vi "daqmx_task output_test.vi"() -> ()   [LabVIEW 2013]
uses:
  <vilib>/DAQmx/read.llb/DAQmx Read (Analog 1D Wfm NChan NSamp).vi
panel:
  out "time string 3":string
  out "time string 2":string
  out "time string":string
  out "error out 2":errorcluster
  out "error out":errorcluster
  out "data 3":waveform(dbl)[](graph) caption="data"
  out "data 2":waveform(dbl)[](graph) caption="data"
  out "data":waveform(dbl)[](graph)
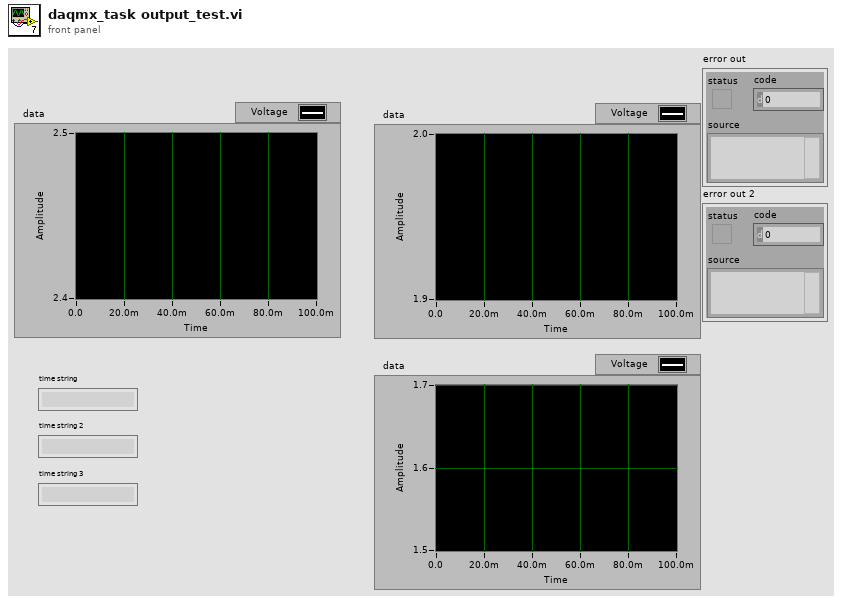
[diagram p1: front panel]
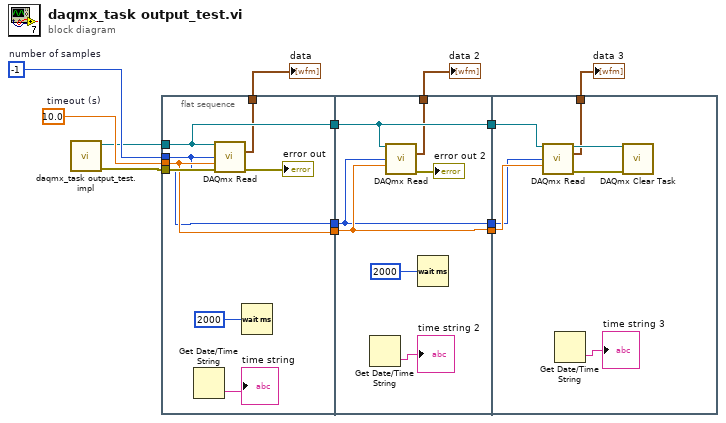
[diagram p0: block diagram]
diagram:
  w12 = 10.0  # timeout (s)
  w13 = -1  # number of samples
  n1 = call "daqmx_task output_test.impl.vi"() -> ("error out"=w10:errorcluster, "task out"=w11:refnum<k21>)  [unwired: 10 in]
  n2 = flat-sequence {
    tunnel: w13 -> [w17]
    tunnel: w12 -> [w18]
    tunnel: w11 -> [w20]
    tunnel: w10 -> [w21]
    tunnel: [w20] -> w9
    tunnel: [w19] -> w7
    tunnel: [w18] -> w4
    tunnel: [w17] -> w2
    tunnel: w9 -> [w28]
    tunnel: [w28] -> w8
    tunnel: [w27] -> w6
    tunnel: w4 -> [w26]
    tunnel: [w26] -> w3
    tunnel: w2 -> [w25]
    tunnel: [w25] -> w1
    tunnel: w8 -> [w33]
    tunnel: [w32] -> w5
    tunnel: w3 -> [w31]
    tunnel: w1 -> [w30]
    frame #0 {
      n3 = Get Date/Time String() -> (time string=→"time string":string)  [unwired: 3 in, 1 out]
      n4 = call-poly <vilib>:"DAQmx Read.vi"("task/channels in"=w20, "number of samples per channel"=w17, "timeout"=w18, "error in"=w21) -> ("data"=w19:waveform(dbl)[], "error out"=→"error out":errorcluster)  [unwired: 9 in, 1 out]
      n5 = Wait (ms)(milliseconds to wait=u32 2000) -> ()  [unwired: 1 out]
    }
    frame #1 {
      n6 = Get Date/Time String() -> (time string=→"time string 2":string)  [unwired: 3 in, 1 out]
      n7 = call-poly <vilib>:"DAQmx Read.vi"("task/channels in"=w28, "number of samples per channel"=w25, "timeout"=w26) -> ("data"=w27:waveform(dbl)[], "error out"=→"error out 2":errorcluster)  [unwired: 10 in, 1 out]
      n8 = Wait (ms)(milliseconds to wait=u32 2000) -> ()  [unwired: 1 out]
    }
    frame #2 {
      n9 = call-poly <vilib>:"DAQmx Read.vi"("task/channels in"=w33, "number of samples per channel"=w30, "timeout"=w31) -> ("task out"=w35:refnum<k21>, "data"=w32:waveform(dbl)[], "error out"=w34:errorcluster)  [unwired: 10 in]
      n10 = Get Date/Time String() -> (time string=→"time string 3":string)  [unwired: 3 in, 1 out]
      n11 = call <vilib>:"DAQmx Clear Task.vi"("task in"=w35, "error in"=w34) -> ()  [unwired: 13 in, 1 out]
    }
  }
  "data" <- w7
  "data 3" <- w5
  "data 2" <- w6
